vi "Init.vi"(11 "Cmd Q":refnum<queue>) -> ()   [LabVIEW 2020, in "FormulaG.lvlib" / "Reset Cmd.lvclass"]
uses:
  Reset Cmd.lvclass
  Command/Command.lvclass
  C:/dev/SummerOfLabVIEW/sol-formulag/ProjectTemplates/Source/SummerOfLabVIEW/FormulaG/template/FormulaG/Command/Command.lvclass
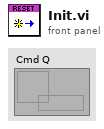
[diagram p1: front panel]
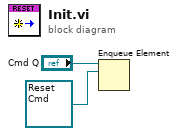
[diagram p0: block diagram]
diagram:
  n1 = Enqueue Element(queue="Cmd Q", element=refnum<class "Reset Cmd.lvclass"> refnum ("FormulaG.lvlib:Reset Cmd.lvclass")) -> ()  [unwired: 2 in, 3 out]
